vi "Elevator Simulator.vi"() -> ()   [LabVIEW 2023]
uses:
  <vilib>/robotics/Kinematics/DH Kinematic Parameters.ctl
  <vilib>/robotics/Kinematics/Link/Joint Type.ctl
  <vilib>/Utility/miscctls.llb/LV3DPointTypeDef.ctl
  <vilib>/robotics/Kinematics/RotateX.vi
  <vilib>/robotics/Kinematics/RotateY.vi
  <vilib>/robotics/Kinematics/RotateZ.vi
  <vilib>/Analysis/baseanly.llb/A x B.vi
  <vilib>/Analysis/baseanly.llb/Real A x B.vi
  <vilib>/picture/3D Picture Control/Object/Create Object (drawable).vi
  <vilib>/picture/3D Picture Control/Object/Add Object (no reference).vi
  <vilib>/robotics/Kinematics/Analytical/Initialize Generic Serial Arm.vi
  <vilib>/robotics/Kinematics/Analytical/NI_Robotics_AnalyticKinematics.lvlib
  <vilib>/robotics/Kinematics/Robot/NI_Robotics_Serial Robot Arm.lvclass
  <vilib>/robotics/Kinematics/NI_Kinematics.lvlib
  <vilib>/picture/3D Picture Control/NI_3D Picture Control.lvlib
  <vilib>/robotics/Kinematics/Plotting/NI_Robotics_3DKinematics.lvlib
  <vilib>/robotics/Kinematics/Link/NI_Robotics_Link.lvclass
panel:
  out "3D Arm Simulation":refnum<vi>(3d-picture)
  in  "Goal End Effector Position":cluster{dbl, dbl, dbl}={0.0, 28.0, 26.0}
  in  "Reset 3D View 2":bool
  in  "Manual Joint Settings":dbl[](array[numeric])=[0.0, 0.0, 0.0, 0.0]
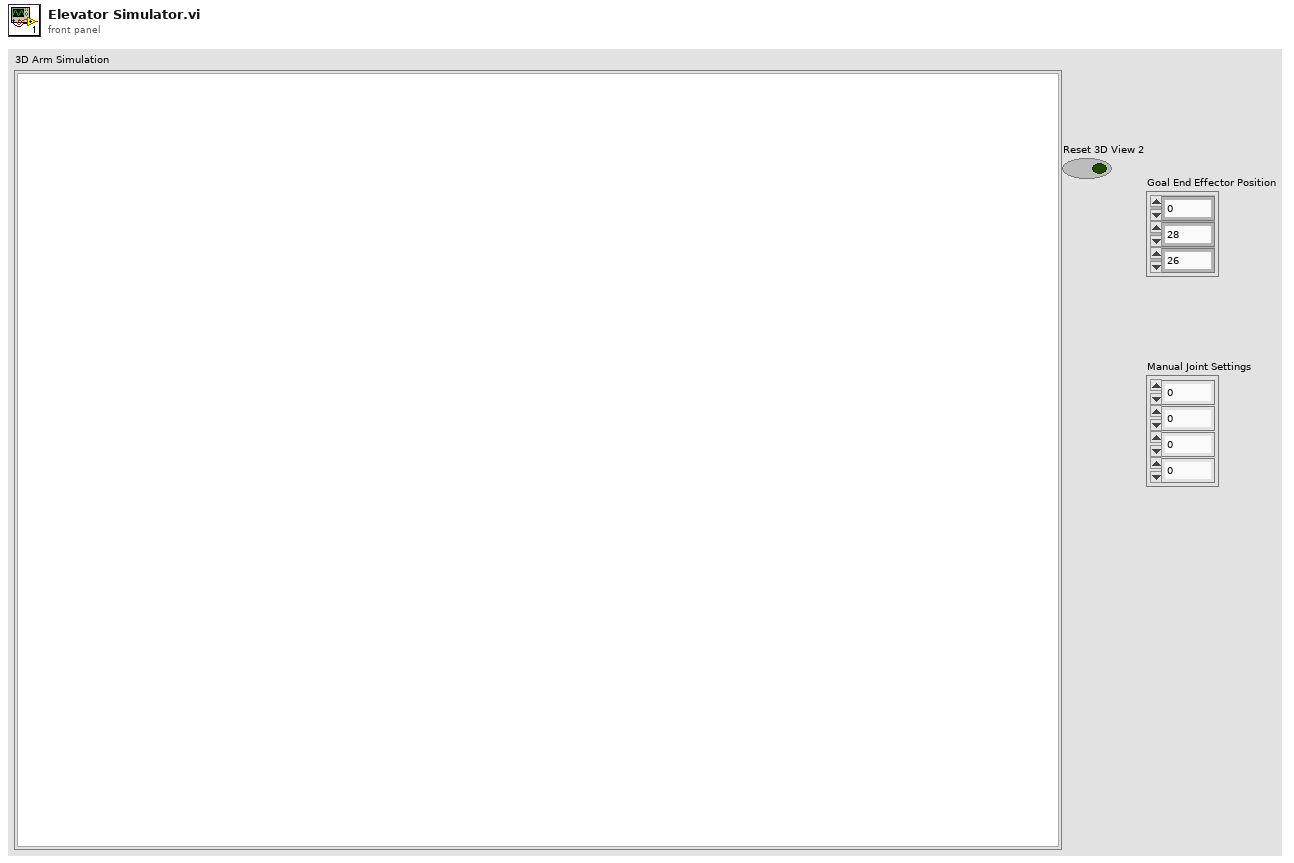
[diagram p1: front panel]
types:
  T1 = cluster{"Red":sgl, "Green":sgl, "Blue":sgl, "Alpha":sgl}
  T2 = typedef "DH Kinematic Parameters.ctl" = cluster{"twist angle":dbl, "length":dbl, "rotation angle":dbl, "offset distance":dbl, "joint type":T3, "joint coordinate offset":dbl}
  T3 = typedef "NI_Robotics_Link.lvclass/Joint Type.ctl" = enum16{"Revolute", "Prismatic"}
  T4 = typedef "NI_Matrix.lvlib/RealMatrix.ctl" = dbl[][]
  T5 = typedef "LV3DPointTypeDef.ctl" = cluster{"X":sgl, "Y":sgl, "Z":sgl}
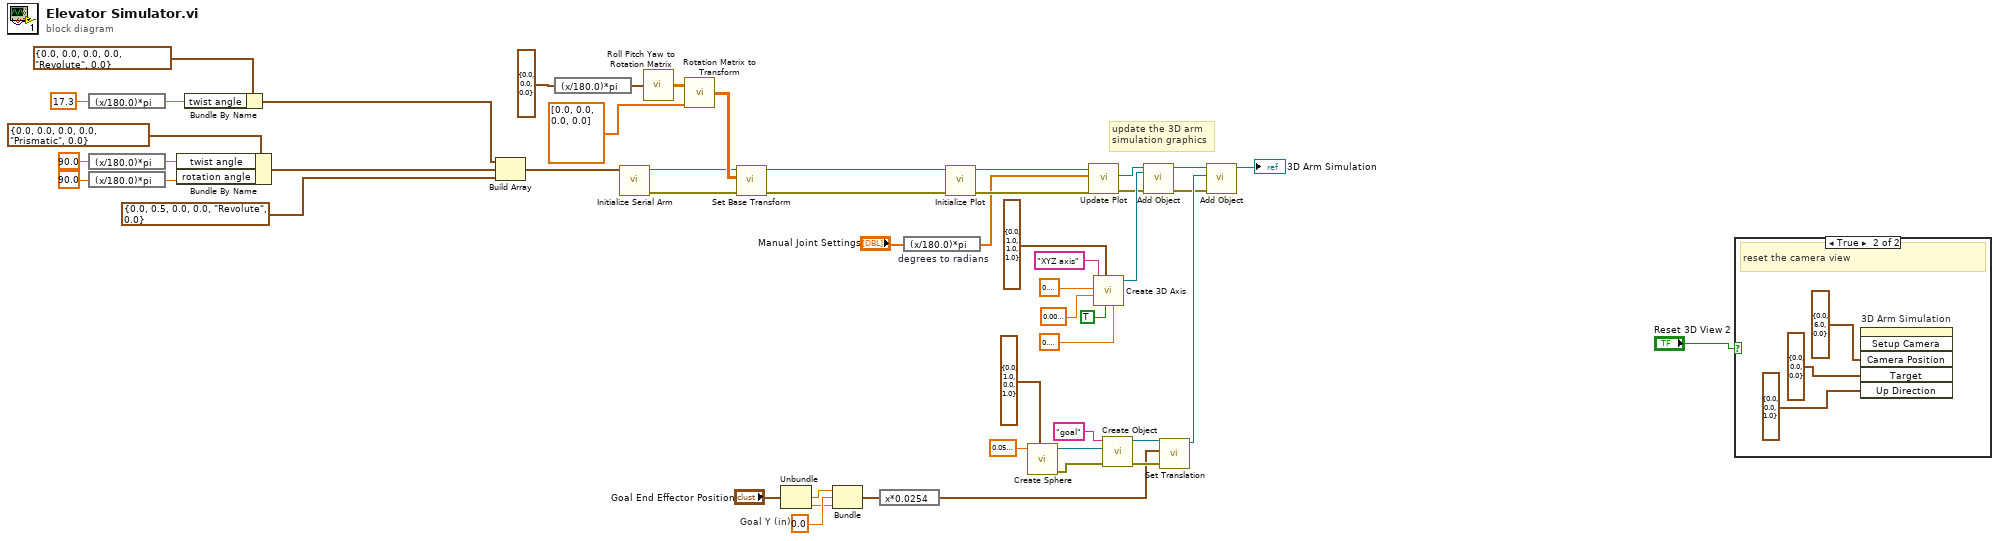
[diagram p0: block diagram]
diagram:
  w17 = 0.0  # Goal Y (in)
  # "update the 3D arm\nsimulation graphics"
  n1 = expression code="(x/180.0)*pi" ("degrees to radians")(17.3 ("twist angle")) -> (w42:dbl)
  n2 = expression code="(x/180.0)*pi" ("degrees to radians")(90.0 ("twist angle")) -> (w8:dbl)
  n3 = expression code="(x/180.0)*pi" ("degrees to radians")(90.0 ("twist angle")) -> (w3:dbl)
  n4 = Bundle By Name(cluster=T2 {"twist angle"=0.0, "length"=0.0, "rotation angle"=0.0, "offset distance"=0.0, "joint type"=enum."Prismatic", "joint coordinate offset"=0.0} ("Link Parameters"), "twist angle"=w8, "rotation angle"=w3) -> (w6:T2)
  n5 = Bundle By Name(cluster=T2 {"twist angle"=0.0, "length"=0.0, "rotation angle"=0.0, "offset distance"=0.0, "joint type"=enum."Revolute", "joint coordinate offset"=0.0} ("Link Parameters"), "twist angle"=w42) -> (w40:T2)
  n6 = Build Array(w40, w6, T2 {"twist angle"=0.0, "length"=0.5, "rotation angle"=0.0, "offset distance"=0.0, "joint type"=enum."Revolute", "joint coordinate offset"=0.0} ("Link Parameters")) -> (w52:T2[])
  n7 = expression code="(x/180.0)*pi" ("degrees to radians")(cluster{"roll":dbl, "pitch":dbl, "yaw":dbl} {"roll"=0.0, "pitch"=0.0, "yaw"=0.0} ("angles")) -> (w48:cluster{"roll":dbl, "pitch":dbl, "yaw":dbl})
  n8 = call-poly <vilib>:"Initialize Serial Arm.vi"("kinematic parameters"=w52) -> ("error out"=w45:errorcluster, "serial arm out"=w47:refnum<class "NI_Robotics_Serial Robot Arm.lvclass">)  [unwired: 9 in]
  n9 = call <vilib>:"Roll Pitch Yaw to Rotation Matrix.vi"("angles"=w48) -> ("rotation matrix"=w49:T4)
  n10 = call <vilib>:"Rotation Matrix to Transform.vi"("translation vector"=dbl[] [0.0, 0.0, 0.0, 0.0] ("Default Value"), "rotation matrix"=w49) -> ("transform"=w50:T4)
  n11 = call <vilib>:"Set Base Transform.vi"("error in (no error)"=w45, "base transform"=w50, "serial arm in"=w47) -> ("error out"=w44:errorcluster, "serial arm out"=w46:refnum<class "NI_Robotics_Serial Robot Arm.lvclass">)  [unwired: 7 in]
  n12 = Unbundle("Goal End Effector Position") -> (w12:dbl, w11:dbl)  [unwired: 1 out]
  n13 = Bundle(w12, "Goal Y (in)"=w17, w11) -> (w16:cluster{dbl, "Goal Y (in)":dbl, dbl})  [unwired: 1 in]
  n14 = expression code="x*0.0254" ("degrees to radians")(w16) -> (w15:cluster{dbl, "Goal Y (in)":dbl, dbl})
  n15 = expression code="(x/180.0)*pi" "degrees to radians"("Manual Joint Settings") -> (w14:dbl[])
  n16 = call <vilib>:"Initialize Plot.vi"("error in (no error)"=w44, "serial arm in"=w46) -> ("error out"=w22:errorcluster, "serial arm out"=w21:refnum<class "NI_Robotics_Serial Robot Arm.lvclass">)  [unwired: 8 in]
  n17 = call <vilib>:"Create Sphere.vi"("Color"=T1 {"Red"=0.0, "Green"=1.0, "Blue"=0.0, "Alpha"=1.0}, "Radius"=sgl 0.05) -> ("error out"=w18:errorcluster, "New Sphere Refnum"=w23:refnum<vi>)  [unwired: 8 in]
  n18 = call <vilib>:"Update Plot.vi"("error in (no error)"=w22, "joint positions"=w14, "serial arm in"=w21) -> ("error out"=w20:errorcluster, "serial arm scene"=w39:refnum<vi>)  [unwired: 6 in, 1 out]
  n19 = call <vilib>:"Create 3D Axis.vi"("Character Size"=sgl 0.1, "Axis label?"=TRUE, "Color"=T1 {"Red"=0.0, "Green"=1.0, "Blue"=1.0, "Alpha"=1.0}, "Radius"=sgl 0.01, "Length"=sgl 0.2, "Name"="XYZ axis") -> ("New Object Refnum"=w32:refnum<vi>)  [unwired: 4 in, 1 out]
  n20 = call-poly <vilib>:"Create Object.vi"("error in (no error)"=w18, "Geometry"=w23, "Name"="goal") -> ("error out"=w29:errorcluster, "Scene:New Object"=w26:refnum<vi>)  [unwired: 7 in]
  n21 = call-poly <vilib>:"Add Object.vi"("error in (no error)"=w20, "New Object In"=w32, "Scene Object In"=w39) -> ("error out"=w19:errorcluster, "Scene Object Out"=w31:refnum<vi>)  [unwired: 7 in]
  n22 = call <vilib>:"Set Translation.vi"("error in (no error)"=w29, "Translation"=w15, "Scene Object"=w26) -> ("Translated Object"=w30:refnum<vi>)  [unwired: 7 in, 1 out]
  n23 = call-poly <vilib>:"Add Object.vi"("error in (no error)"=w19, "New Object In"=w30, "Scene Object In"=w31) -> ("Scene Object Out"=→"3D Arm Simulation":refnum<vi>)  [unwired: 7 in, 1 out]
  n24 = case shown="True" "Reset 3D View 2" {
    frame False {
    }
    frame True {
      # "reset the camera view"
      n25 = invoke on="3D Arm Simulation" class="SceneGraphDisp (strict)" method="Setup Camera"("Camera Position"=T5 {"X"=0.0, "Y"=6.0, "Z"=0.0}, "Target"=T5 {"X"=0.0, "Y"=0.0, "Z"=0.0}, "Up Direction"=T5 {"X"=0.0, "Y"=0.0, "Z"=1.0}) -> ()  [unwired: 3 in, 6 out]
    }
  }
